vi "用户列表.vi"() -> ()   [LabVIEW 2016, in "Alarm interface.lvlib" / "短信语音库.lvlib"]
uses:
  <vilib>/Utility/miscctls.llb/LVPointTypeDef.ctl
  Alarm interface.lvlib
panel:
  in  "修改":bool
  in  "关闭":bool
  in  "删除":bool
  in  "添加":bool
  in  "短信语音用户列表":i32(listbox)
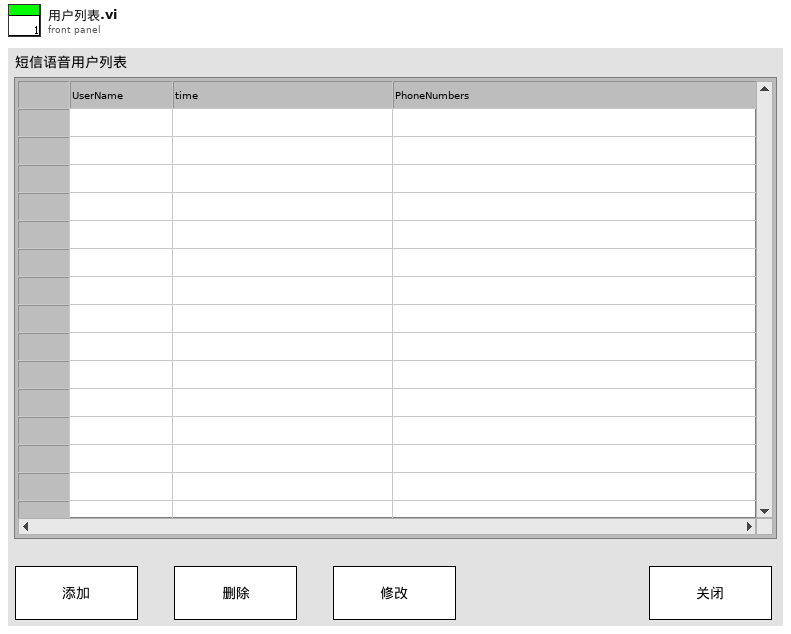
[diagram p1: front panel]
types:
  T1 = typedef "LVPointTypeDef.ctl" = cluster{"Horizontal":i16, "Vertical":i16}
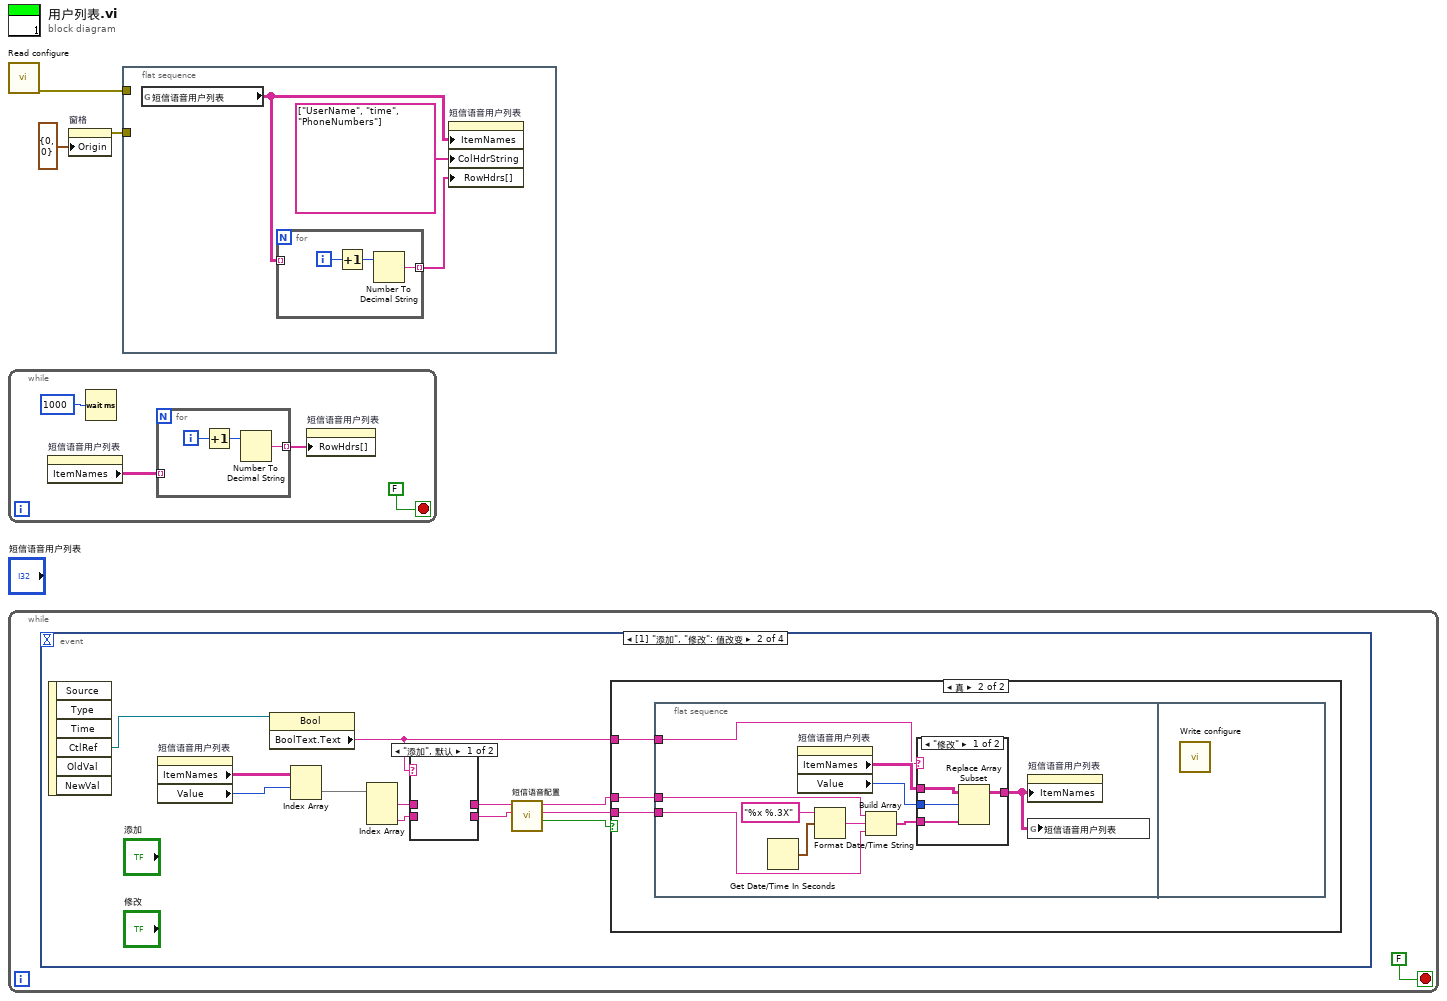
[diagram p0: block diagram]
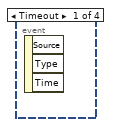
[diagram p2: hidden frame]
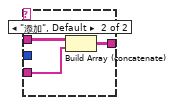
[diagram p5: hidden frame]
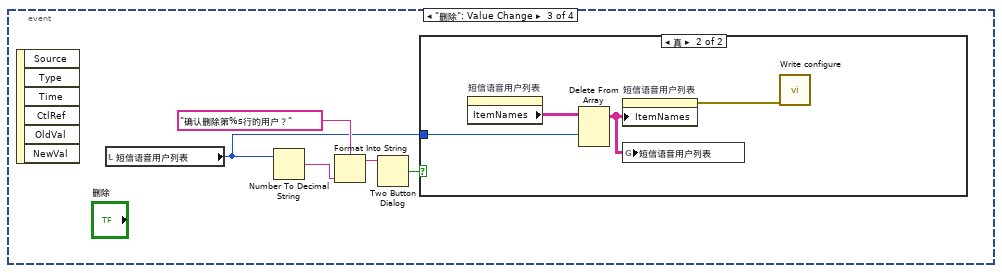
[diagram p6: hidden frame]
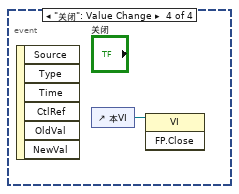
[diagram p8: hidden frame]
diagram:
  n1 = call "Read configure.vi"() -> ("error out"=w1:errorcluster)  [unwired: 11 in]
  n2 = while {
    stop <- FALSE stop-if-true
    n3 = property on="短信语音用户列表" class="MCListbox (严格)"() -> ("ItemNames"=w5:string[][])  [unwired: 2 in, 2 out]
    n4 = Wait (ms)(milliseconds to wait=u32 1000 ("等待时间（毫秒）")) -> ()  [unwired: 1 out]
    n5 = for {
      tunnel: [w9] -> w4 mode=indexing
      tunnel: w5 -> [_] mode=indexing
      i -> [w10]
      n6 = Increment(x=w10) -> (x+1=w8:i32)
      n7 = Number To Decimal String(number=w8) -> (decimal integer string=w9:string)  [unwired: 1 in]
    }
    n8 = property on="短信语音用户列表" class="MCListbox (严格)"("RowHdrs[]"=w4) -> ()  [unwired: 2 in, 2 out]
  }
  n9 = while {
    stop <- FALSE stop-if-true
    n10 = event shown="[1] \"添加\", \"修改\": 值改变" {
      selector: _ -> [_ _ _ _]
      dyn-events: _ -> [_ _ _ _]
      timeout: _ -> [_ _ _ _]
      event Timeout {
        n11 = event-data() -> ()  [unwired: 1 in, 3 out]
      }
      event "添加", "修改": Value Change {
        n12 = event-data() -> ("CtlRef"=w20:refnum<vi>)  [unwired: 1 in, 5 out]
        n13 = property on="短信语音用户列表" class="MCListbox (严格)"() -> ("ItemNames"=w19:string[][], "Value"=w18:i32)  [unwired: 2 in, 2 out]
        n14 = property class="Bool"(reference=w20) -> ("BoolText.Text"=w12:string)  [unwired: 1 in, 2 out]
        n15 = Index Array(array=w19, index (row)=w18) -> (element=w17:string[])  [unwired: 1 in]
        n16 = Index Array(array=w17) -> (element #1=w16:string, element #3=w15:string)  [unwired: 3 in, 1 out]
        n17 = case shown="\"添加\", 默认" w12 {
          tunnel: w16 -> [_ w25]
          tunnel: w15 -> [_ w24]
          tunnel: [_ w25] -> w14
          tunnel: [_ w24] -> w13
          frame "添加", Default {
          }
          frame "修改" {
          }
        }
        n18 = call "短信语音配置.vi"("电话"=w13, "姓名"=w14) -> ("输出"=w21:bool, "电话输出"=w22:string, "姓名输出"=w23:string)  [unwired: 7 in]
        n19 = case shown="真" w21 {
          tunnel: w23 -> [_ w28]
          tunnel: w22 -> [_ w27]
          tunnel: w12 -> [_ w26]
          frame False {
          }
          frame True {
            n20 = flat-sequence {
              tunnel: w28 -> [w36]
              tunnel: w27 -> [w34]
              tunnel: w26 -> [w30]
              frame #0 {
                n21 = Get Date/Time In Seconds() -> (seconds since 1Jan1904=w37:timestamp)
                n22 = property on="短信语音用户列表" class="MCListbox (严格)"() -> ("ItemNames"=w33:string[][], "Value"=w29:i32)  [unwired: 2 in, 2 out]
                n23 = Format Date/Time String(time format string (%c)="%x %.3X" ("时间格式字符串(%c)"), seconds (now)=w37) -> (date/time string=w35:string)  [unwired: 1 in]
                n24 = Build Array(w36, w35, w34) -> (w32:string[])
                n25 = case shown="\"修改\"" w30 {
                  tunnel: w33 -> [w42 w45]
                  tunnel: w32 -> [w41 w44]
                  tunnel: [w39 w43] -> w31
                  tunnel: w29 -> [w40 _]
                  frame "修改" {
                    n26 = Replace Array Subset(array=w42, new element=w41, index (row)=w40) -> (w39:string[][])  [unwired: 1 in]
                  }
                  frame "添加", Default {
                    n27 = Build Array (concatenate)(w45, w44) -> (w43:string[][])
                  }
                }
                n28 = property on="短信语音用户列表" class="MCListbox (严格)"("ItemNames"=w31) -> ()  [unwired: 2 in, 2 out]
                n29 = global write "断电保存全局.vi" "短信语音用户列表"(w31) -> ()
              }
              frame #1 {
                n30 = call "Write configure.vi"() -> ()  [unwired: 11 in, 1 out]
              }
            }
          }
        }
      }
      event "删除": Value Change {
        n31 = event-data() -> ()  [unwired: 1 in, 6 out]
        n32 = local read "短信语音用户列表"() -> (w49:i32)
        n33 = Number To Decimal String(number=w49) -> (decimal integer string=w48:string)  [unwired: 1 in]
        n34 = Format Into String(format string="确认删除第%s行的用户？" ("消息"), w48) -> (resulting string=w47:string)  [unwired: 2 in, 1 out]
        n35 = Two Button Dialog(message=w47) -> (T button?=w46:bool)  [unwired: 2 in]
        n36 = case shown="真" w46 {
          tunnel: w49 -> [_ w53]
          frame False {
          }
          frame True {
            n37 = property on="短信语音用户列表" class="MCListbox (严格)"() -> ("ItemNames"=w54:string[][])  [unwired: 2 in, 2 out]
            n38 = Delete From Array(array=w54, index (row)=w53) -> (array with subset deleted=w52:string[][])  [unwired: 2 in, 1 out]
            n39 = property on="短信语音用户列表" class="MCListbox (严格)"("ItemNames"=w52) -> (error out=w51:errorcluster)  [unwired: 2 in, 1 out]
            n40 = global write "断电保存全局.vi" "短信语音用户列表"(w52) -> ()
            n41 = call "Write configure.vi"("error in (no error)"=w51) -> ()  [unwired: 10 in, 1 out]
          }
        }
      }
      event "关闭": Value Change {
        n42 = event-data() -> ()  [unwired: 1 in, 6 out]
        n43 = control-ref of="本VI"() -> (w55:refnum<vi>)
        n44 = invoke class="VI" method="FP.Close"(reference=w55) -> ()  [unwired: 2 in, 3 out]
      }
    }
  }
  n45 = property on="窗格" class="Pane"("Origin"=T1 {"Horizontal"=0, "Vertical"=0} ("原点")) -> (error out=w2:errorcluster)  [unwired: 2 in, 1 out]
  n46 = flat-sequence {
    tunnel: w2 -> [_]
    tunnel: w1 -> [_]
    frame #0 {
      n47 = global read "断电保存全局.vi" "短信语音用户列表"() -> (w57:string[][])
      n48 = for {
        tunnel: w57 -> [_] mode=indexing
        tunnel: [w60] -> w56 mode=indexing
        i -> [w61]
        n49 = Increment(x=w61) -> (x+1=w59:i32)
        n50 = Number To Decimal String(number=w59) -> (decimal integer string=w60:string)  [unwired: 1 in]
      }
      n51 = property on="短信语音用户列表" class="MCListbox (严格)"("ItemNames"=w57, "ColHdrString"=string[] ["UserName", "time", "PhoneNumbers"] ("列首字符串[]"), "RowHdrs[]"=w56) -> ()  [unwired: 2 in, 2 out]
    }
  }
